vi "Side Actuators.vi"(9 "Boolean":bool=TRUE, 11 "Input":T1) -> (2 "Output Cmd":dbl)   [LabVIEW 2009]
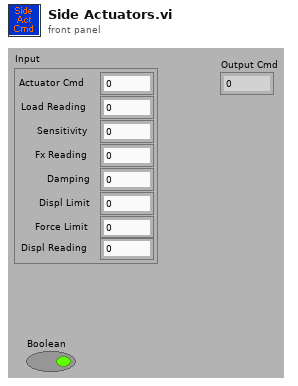
[diagram p1: front panel]
types:
  T1 = cluster{"Actuator Cmd":dbl, "Load Reading":dbl, "Sensitivity":dbl, "Fx Reading":dbl, "Damping":dbl, "Displ Limit":dbl, "Force Limit":dbl, "Displ Reading":dbl}
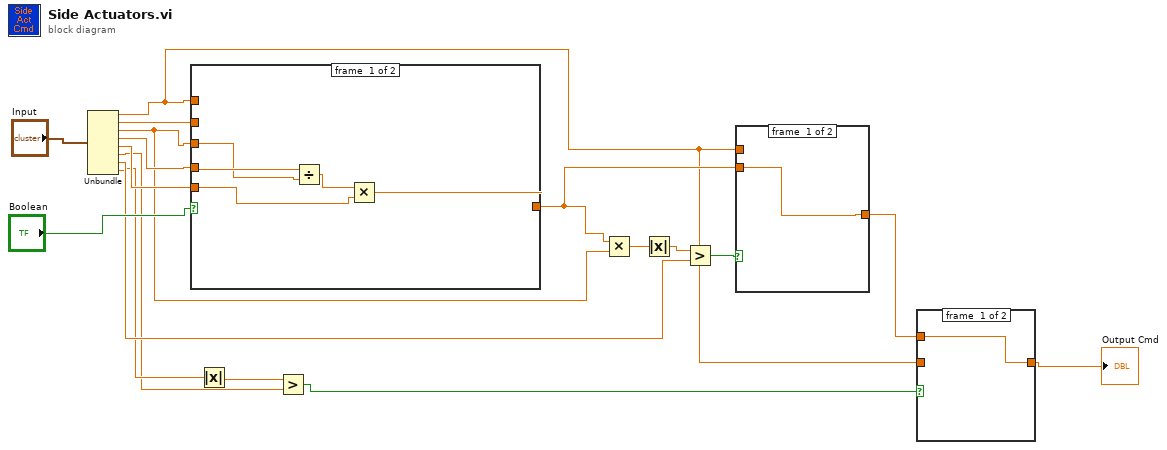
[diagram p0: block diagram]
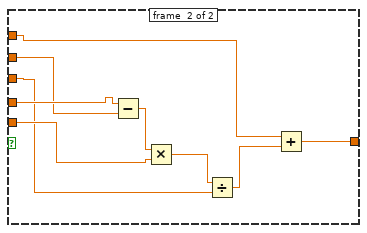
[diagram p4: hidden frame]
diagram:
  n1 = Unbundle("Input") -> ("Actuator Cmd"=w2:dbl, "Load Reading"=w16:dbl, "Sensitivity"=w13:dbl, "Fx Reading"=w15:dbl, "Damping"=w14:dbl, "Displ Limit"=w5:dbl, "Force Limit"=w10:dbl, "Displ Reading"=w7:dbl)
  n2 = case shown="True" "Boolean" {
    tunnel: w2 -> [_ w25]
    tunnel: w16 -> [_ w31]
    tunnel: w13 -> [w22 w28]
    tunnel: w15 -> [w23 w32]
    tunnel: w14 -> [w21 w29]
    tunnel: [w19 w24] -> w8
    frame #0 {
      n3 = Divide(x=w23, y=w22) -> (x/y=w20:dbl)
      n4 = Multiply(x=w20, y=w21) -> (x*y=w19:dbl)
    }
    frame #1 {
      n5 = Subtract(x=w32, y=w31) -> (x-y=w30:dbl)
      n6 = Multiply(x=w30, y=w29) -> (x*y=w27:dbl)
      n7 = Divide(x=w27, y=w28) -> (x/y=w26:dbl)
      n8 = Add(x=w25, y=w26) -> (x+y=w24:dbl)
    }
  }
  n9 = Absolute Value(x=w7) -> (abs(x)=w6:dbl)
  n10 = Greater?(x=w6, y=w5) -> (0:w4:bool)
  n11 = Multiply(x=w8, y=w13) -> (x*y=w12:dbl)
  n12 = Absolute Value(x=w12) -> (abs(x)=w11:dbl)
  n13 = Greater?(x=w11, y=w10) -> (0:w9:bool)
  n14 = case shown="False" w9 {
    tunnel: w2 -> [_ w34]
    tunnel: w8 -> [w33 _]
    tunnel: [w33 w34] -> w3
    frame #0 {
    }
    frame #1 {
    }
  }
  n15 = case shown="False" w4 {
    tunnel: w3 -> [w35 _]
    tunnel: w2 -> [_ w36]
    tunnel: [w35 w36] -> w1
    frame #0 {
    }
    frame #1 {
    }
  }
  "Output Cmd" <- w1
